vi "01. LoginDlg.vi"(11 "password":string) -> (3 "login ok?":bool)   [LabVIEW 2018]
uses:
  Module/Library-Ctrl/Library-Ctrl.lvlib
panel:
  in  "cancel btn":bool
  in  "login btn":bool
  in  "input":string caption="PASSWORD"
  # "관리자 로그인"
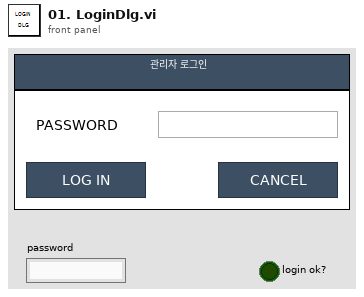
[diagram p1: front panel]
types:
  T1 = typedef "eventvkey.ctl" = enum16{"ASCII", "Enter", "Return", "Shift", "Ctrl", "Alt", "Cmd", "Opt", "Caps", "NumLock", "Clear", "Break", "Up", "Down", "Left", "Right", "Insert", "Delete", "Home", "End", "PageUp", "PageDown", "Escape", "Help", "Pause", "ScrollLock", "F1", "F2", "F3", "F4", "F5", "F6", "F7", "F8", "F9", "F10", "F11", "F12", "F13", "F14", "F15", "F16", "F17", "F18", "F19", "F20", "F21", "F22", "F23", "F24", "Play", "VolumeUp", "VolumeDown", "Mute", "Two Byte Char"}
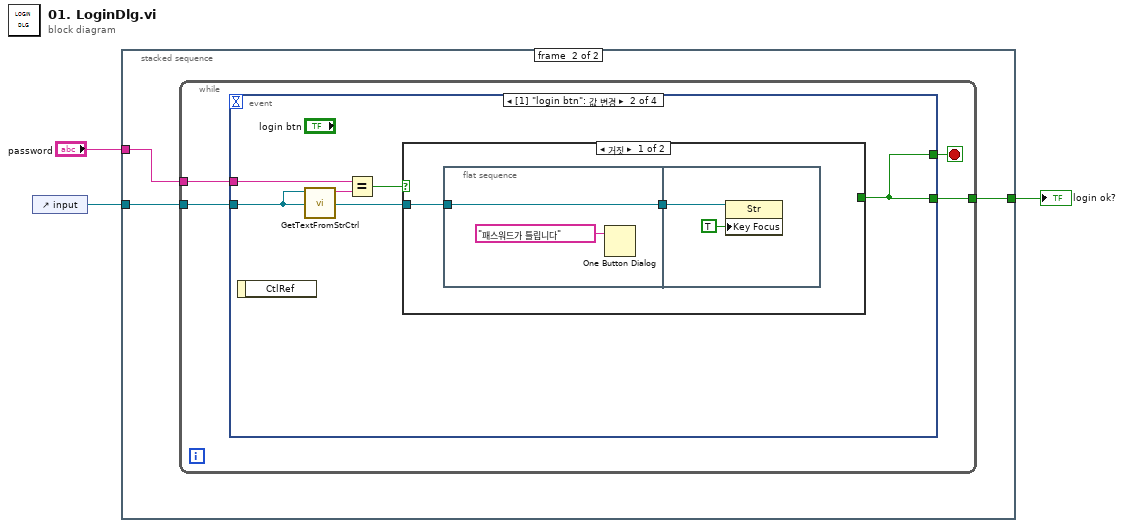
[diagram p0: block diagram]
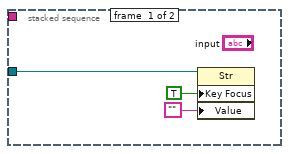
[diagram p2: hidden frame]
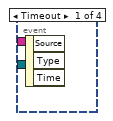
[diagram p3: hidden frame]
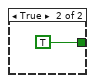
[diagram p4: hidden frame]
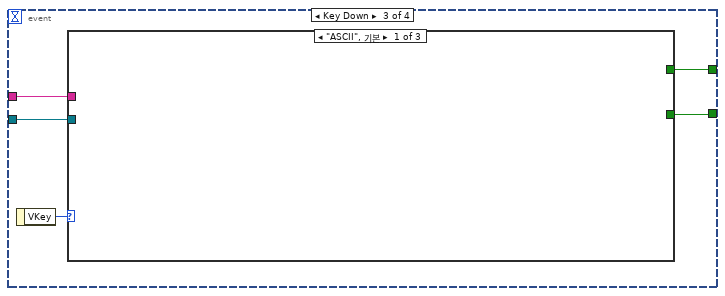
[diagram p5: hidden frame]
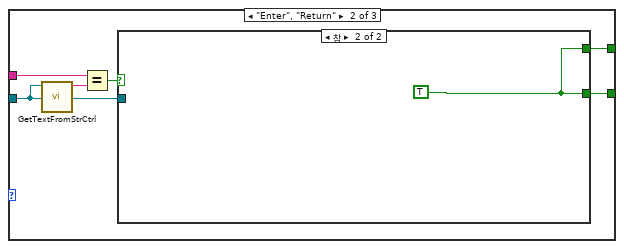
[diagram p6: hidden frame]
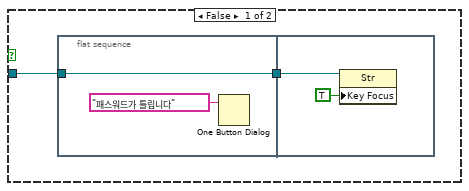
[diagram p7: hidden frame]
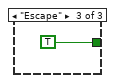
[diagram p8: hidden frame]
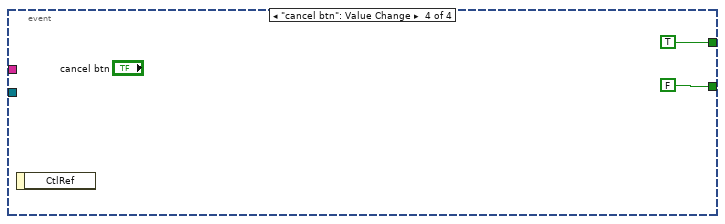
[diagram p9: hidden frame]
diagram:
  n1 = control-ref of="input"() -> (w1:refnum<vi>)
  n2 = stacked-sequence {
    tunnel: [_ w9] -> w3
    tunnel: "password" -> [_ w7]
    tunnel: w1 -> [w4 w8]
    frame #0 {
      n3 = property class="Str"(reference=w4, "Key Focus"=TRUE ("키 포커스"), "Value"="") -> ()  [unwired: 1 in, 2 out]
    }
    frame #1 {
      n4 = while {
        tunnel: [w12] -> w9
        tunnel: w7 -> [w11]
        tunnel: w8 -> [w10]
        stop <- w13 stop-if-true
        n5 = event shown="[1] \"login btn\": 값 변경" {
          selector: _ -> [_ _ _ _]
          dyn-events: _ -> [_ _ _ _]
          timeout: _ -> [_ _ _ _]
          tunnel: [_ w16 w26 TRUE] -> w13
          tunnel: [_ w16 w27 FALSE] -> w12
          tunnel: w11 -> [_ w18 w29 _]
          tunnel: w10 -> [_ w14 w28 _]
          event Timeout {
            n6 = event-data() -> ()  [unwired: 1 in, 3 out]
          }
          event "login btn": Value Change {
            n7 = event-data() -> ()  [unwired: 1 in, 1 out]
            n8 = call "GetTextFromStrCtrl.vi"("string ref"=w14) -> ("string out"=w15:string)  [unwired: 10 in]
            n9 = Equal?(x=w18, y=w15) -> (x = y?=w17:bool)
            n10 = case shown="거짓" w17 {
              tunnel: [_ TRUE] -> w16
              tunnel: w14 -> [w20 _]
              frame False {
                n11 = flat-sequence {
                  tunnel: w20 -> [w22]
                  tunnel: [w22] -> w19
                  tunnel: w19 -> [w23]
                  frame #0 {
                    n12 = One Button Dialog(message="패스워드가 틀립니다" ("메시지")) -> ()  [unwired: 1 in, 1 out]
                  }
                  frame #1 {
                    n13 = property class="Str"(reference=w23, "Key Focus"=TRUE ("키 포커스")) -> ()  [unwired: 1 in, 2 out]
                  }
                }
              }
              frame True {
              }
            }
          }
          event Key Down {
            n14 = event-data() -> ("VKey"=w30:T1)  [unwired: 1 in]
            n15 = case shown="\"ASCII\", 기본" w30 {
              tunnel: w29 -> [_ w35 _]
              tunnel: w28 -> [_ w32 _]
              tunnel: [_ w33 _] -> w27
              tunnel: [_ w31 TRUE] -> w26
              frame "ASCII", Default {
              }
              frame "Enter", "Return" {
                n16 = call "GetTextFromStrCtrl.vi"("string ref"=w32) -> ("string out"=w36:string)  [unwired: 10 in]
                n17 = Equal?(x=w35, y=w36) -> (x = y?=w34:bool)
                n18 = case shown="참" w34 {
                  tunnel: [_ w43] -> w33
                  tunnel: w32 -> [w37 _]
                  tunnel: [_ w43] -> w31
                  frame False {
                    n19 = flat-sequence {
                      tunnel: w37 -> [w40]
                      tunnel: [w40] -> w38
                      tunnel: w38 -> [w41]
                      frame #0 {
                        n20 = One Button Dialog(message="패스워드가 틀립니다" ("메시지")) -> ()  [unwired: 1 in, 1 out]
                      }
                      frame #1 {
                        n21 = property class="Str"(reference=w41, "Key Focus"=TRUE ("키 포커스")) -> ()  [unwired: 1 in, 2 out]
                      }
                    }
                  }
                  frame True {
                    w43 = TRUE
                  }
                }
              }
              frame "Escape" {
              }
            }
          }
          event "cancel btn": Value Change {
            n22 = event-data() -> ()  [unwired: 1 in, 1 out]
          }
        }
      }
    }
  }
  "login ok?" <- w3
